vi "Analog DAQ_Read.vi"(0 "Analog DAQ In":refnum<class "Analog DAQ.lvclass">, 11 "error in (no error)":errorcluster) -> (4 "Analog DAQ Out":refnum<class "Analog DAQ.lvclass">, 8 "Current Value":dbl format="%0.2f", 15 "error out":errorcluster)   [LabVIEW 2013, in "Analog DAQ.lvclass"]
uses:
  Analog DAQ.lvclass
  Actor/src/Connector/FTW-ActorConnector.lvclass
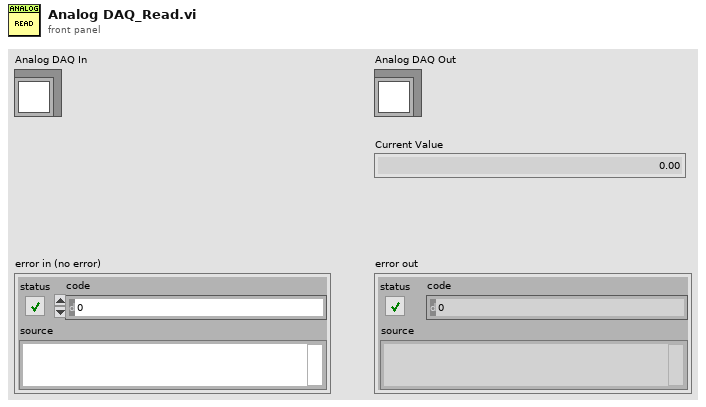
[diagram p1: front panel]
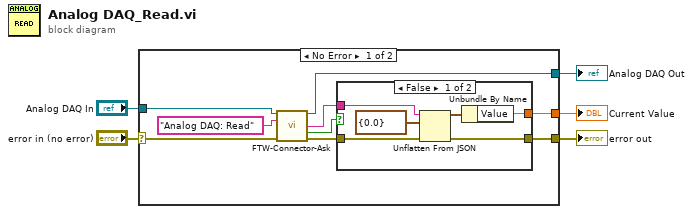
[diagram p0: block diagram]
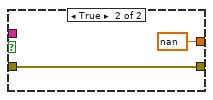
[diagram p2: hidden frame]
diagram:
  n1 = case shown="No Error" "error in (no error)" {
    selector: "error in (no error)" -> [w12 w23]
    tunnel: "Analog DAQ In" -> [w14 w24]
    tunnel: [w13 w24] -> w3
    tunnel: [w9 w23] -> w2
    tunnel: [w7 _] -> w1
    frame No Error {
      n2 = call "FTW-Connector-Ask.vi"("FTW Actor Connector"=w14, "Request Header"="Analog DAQ: Read", "error in"=w12) -> ("FTW Actor Connector out"=w13:refnum<class "Analog DAQ.lvclass">, "Response Body"=w8:string, "Timed out?"=w6:bool, "error out"=w11:errorcluster)  [unwired: 7 in, 2 out]
      n3 = case shown="False" w6 {
        tunnel: w11 -> [w20 w22]
        tunnel: [w19 w22] -> w9
        tunnel: w8 -> [w18 _]
        tunnel: [w15 nan ("Value")] -> w7
        frame False {
          n4 = Unflatten From JSON(JSON string=w18, type and defaults=cluster{"Value":dbl} {"Value"=0.0}, error in (no error)=w20) -> (value=w16:cluster{"Value":dbl}, error out=w19:errorcluster)  [unwired: 4 in]
          n5 = Unbundle By Name(w16) -> ("Value"=w15:dbl)
        }
        frame True {
        }
      }
    }
    frame Error {
    }
  }
  "Analog DAQ Out" <- w3
  "error out" <- w2
  "Current Value" <- w1
